vi "SPCSetUpToUserInput.vi"(8 "ErrorIn":errorcluster, 11 "SetUp":string="*SETUP\r\n  SYS_PARA_BEGIN:\r\n  #PR [PR_PDEV,I,2]\r\n  #PR [PR_PPORT,I,2]\r\n  #PR [PR_PWHAT,I,1]\r\n  #PR [PR_PF,B,0]\r\n  #PR [PR_PFNAME,S,C:\\Program Files (x86)\\BH\\SPCM\\IMAGE.PRT]\r\n  #PR [PR_PORIEN,I,1]\r\n  #PR [PR_PEJECT,B,1]\r\n  #PR [PR_PWIDTH,F,100]\r\n  #PR [PR_PHEIGH,F,100]\r\n  #PR [PR_PFULL,B,1]\r\n  #PR [PR_PAUTO,B,1]\r\n  #PR [PR_STP_FN,S,C:\\Users\\frank\\Documents\\BHdata\\SPCM\\STP.CFG]\r\n  #PR [PR_SAVE_T,I,0]\r\n  #PR [PR_SLEEP,I,9]\r\n  #SP [SP_MODE,I,11]\r\n  #SP [SP_CFD_LL,F,-29.411764]\r\n  #SP [SP_CFD_LH,F,5.019608]\r\n  #SP [SP_CFD_ZC,F,-5.2913384]\r\n  #SP [SP_CFD_HF,F,5]\r\n  #SP [SP_SYN_ZC,F,-5.2913384]\r\n  #SP [SP_SYN_FD,I,1]\r\n  #SP [SP_SYN_FQ,F,-50.980392]\r\n  #SP [SP_SYN_HF,F,4]\r\n  #SP [SP_TAC_R,F,5.0033574e-08]\r\n  #SP [SP_TAC_G,I,1]\r\n  #SP [SP_TAC_OF,F,0]\r\n  #SP [SP_TAC_LL,F,0]\r\n  #SP [SP_TAC_LH,F,100]\r\n  #SP [SP_TAC_TC,F,1.2215228e-11]\r\n  #SP [SP_TAC_TD,F,5.0033573e-09]\r\n  #SP [SP_ADC_RE,I,4096]\r\n  #SP [SP_EAL_DE,I,0]\r\n  #SP [SP_NCX,I,1]\r\n  #SP [SP_NCY,I,1]\r\n  #SP [SP_PAGE,I,1]\r\n  #SP [SP_COL_T,F,10]\r\n  #SP [SP_REP_T,F,10]\r\n  #SP [SP_DIS_T,F,1]\r\n  #SP [SP_REPEAT,B,0]\r\n  #SP [SP_STOPT,B,1]\r\n  #SP [SP_OVERFL,C,N]\r\n  #SP [SP_WL_STA,F,500]\r\n  #SP [SP_WL_STO,F,551.09998]\r\n  #SP [SP_WL_STE,F,0.1]\r\n  #SP [SP_EXTST,B,0]\r\n  #SP [SP_STEPS,I,64]\r\n  #SP [SP_OFFSET,F,0]\r\n  #SP [SP_YWIN_N,I,8]\r\n  #SP [SP_XWIN_N,I,8]\r\n  #SP [SP_TWIN_N,I,1]\r\n  #SP [SP_X_EQU,B,1]\r\n  #SP [SP_Y_EQU,B,1]\r\n  #SP [SP_T_EQU,B,1]\r\n  #SP [SP_DITH,I,128]\r\n  #SP [SP_EN_INT,B,0]\r\n  #SP [SP_INCR,I,1]\r\n  #SP [SP_DAES,B,0]\r\n  #SP [SP_SPE_FN,S,c:\\Users\\jannis\\Desktop\\SPC file example\\v1.spc]\r\n  #SP [SP_CYCLES,U,1]\r\n  #SP [SP_DAEC,B,1]\r\n  #SP [SP_MEM_BANK,I,0]\r\n  #SP [SP_DTCOMP,B,0]\r\n  #SP [SP_SCF,I,0]\r\n  #SP [SP_POL_L,I,0]\r\n  #SP [SP_POL_F,I,0]\r\n  #SP [SP_PIX,I,0]\r\n  #SP [SP_LDIV,I,0]\r\n  #SP [SP_ACCUM,B,0]\r\n  #SP [SP_ROUT,B,1792]\r\n  #SP [SP_TAC_EH,F,10]\r\n  #SP [SP_DLIM,I,10240000]\r\n  #SP [SP_PHOT_F,U,473956351]\r\n  #SP [SP_EN_DLIM,B,1]\r\n  #SP [SP_PH_BUF,I,65536]\r\n  #SP [SP_FLB_Y,I,1]\r\n  #SP [SP_FLB_X,I,1]\r\n  #SP [SP_BORD_U,I,1]\r\n  #SP [SP_BORD_L,I,1]\r\n  #SP [SP_POL_P,I,1]\r\n  #SP [SP_PIX_T,F,2.1e-05]\r\n  #SP [SP_PIX_CLK,I,1]\r\n  #SP [SP_TRIGGER,I,16]\r\n  #SP [SP_SCAN_X,I,1]\r\n  #SP [SP_SCAN_Y,I,1]\r\n  #SP [SP_SCAN_RX,I,1]\r\n  #SP [SP_SCAN_RY,I,1]\r\n  #SP [SP_FIF_TYP,I,0]\r\n  #SP [SP_EPX_DIV,I,1]\r\n  #SP [SP_MTCLK,I,0]\r\n  #SP [SP_ADD_SEL,I,0]\r\n  #SP [SP_SXWIN_N,I,1]\r\n  #SP [SP_SYWIN_N,I,1]\r\n  #SP [SP_SX_EQU,B,1]\r\n  #SP [SP_SY_EQU,B,1]\r\n  #SP [SP_ASAVE,I,34]\r\n  #SP [SP_ADC_ZOOM,I,0]\r\n  #SP [SP_FIF_FNO,I,1]\r\n  #SP [SP_FCYCLES,U,1]\r\n  #SP [SP_XY_GAIN,I,1]\r\n  #SP [SP_IMG_X,I,512]\r\n  #SP [SP_IMG_Y,I,512]\r\n  #SP [SP_IMG_RX,I,1]\r\n  #SP [SP_IMG_RY,I,1]\r\n  #SP [SP_MST_CLK,I,0]\r\n  #SP [SP_ADC_DE,I,0]\r\n  #SP [SP_DET_TYP,I,0]\r\n  #SP [SP_X_AXIS,I,0]\r\n  #SP [SP_CH_EN,I,4191231]\r\n  #SP [SP_CH_SL,I,16777215]\r\n  #SP [SP_CH_F1,I,0]\r\n  #SP [SP_CH_F2,I,136314880]\r\n  #DI [DI_SCALE,I,0]\r\n  #DI [DI_MAXCNT,L,2]\r\n  #DI [DI_LBLINE,L,1]\r\n  #DI [DI_BLINE,L,0]\r\n  #DI [DI_GRID,B,1]\r\n  #DI [DI_GCOL_F,I,14737632]\r\n  #DI [DI_GCOL_B,I,16777215]\r\n  #DI [DI_TRACE,I,0]\r\n  #DI [DI_BOD_C,I,32896]\r\n  #DI [DI_2DDIS,I,0]\r\n  #DI [DI_2DTRNO,I,1]\r\n  #DI [DI_3DOFFX,I,3]\r\n  #DI [DI_3DOFFY,I,1]\r\n  #DI [DI_3DINCX,I,0]\r\n  #DI [DI_3DCOL,I,0]\r\n  #DI [DI_3DMODE,I,2]\r\n  #DI [DI_YWIN,I,1]\r\n  #DI [DI_XWIN,I,1]\r\n  #DI [DI_TWIN,I,1]\r\n  #DI [DI_PSTYLE,I,1]\r\n  #DI [DI_PFREQ,I,1]\r\n  #DI [DI_CUR,B,0]\r\n  #DI [DI_RATE,B,1]\r\n  #DI [DI_2DC1,B,1]\r\n  #DI [DI_2DC2,B,1]\r\n  #DI [DI_2DC1C,I,10]\r\n  #DI [DI_2DC2C,I,13]\r\n  #DI [DI_2DC1S,I,0]\r\n  #DI [DI_2DC2S,I,0]\r\n  #DI [DI_3DC1C,I,12]\r\n  #DI [DI_3DC2C,I,14]\r\n  #DI [DI_SIZE,I,0]\r\n  #DI [DI_3DSTYL,I,1]\r\n  #DI [DI_INTCOL,I,1]\r\n  #DI [DI_INTPIX,I,1]\r\n  #DI [DI_COL_NO,I,2]\r\n  #DI [DI_COLMIN,I,0]\r\n  #DI [DI_COLMAX,I,16777215]\r\n  #DI [DI_COL2,I,16711680]\r\n  #DI [DI_COL3,I,255]\r\n  #DI [DI_COL4,I,16776960]\r\n  #DI [DI_COL5,I,65280]\r\n  #DI [DI_HICOL,I,16711680]\r\n  #DI [DI_XREV,B,0]\r\n  #DI [DI_YREV,B,0]\r\n  #DI [DI_DETAIL,B,1]\r\n  #DI [DI_SYWIN,I,1]\r\n  #DI [DI_SXWIN,I,1]\r\n  #DI [DI_ASCALE,I,1]\r\n  SYS_PARA_END:\r\n  TRACE_PARA_BEGIN:\r\n  #TR #0 [1,255,1,1,3,1,1,1]1,1,1]\r\n  #TR #1 [0,16711680,1,1,1,2,1,1]1,1,1]\r\n  #TR #2 [0,65280,1,1,1,3,1,1]1,1,1]\r\n  #TR #3 [0,44,1,1,1,4,1,1]1,1,1]\r\n  #TR #4 [0,16718521,1,1,1,1,1,1]1,1,1]\r\n  #TR #5 [0,16765696,1,1,1,1,1,1]1,1,1]\r\n  #TR #6 [0,22528,1,1,1,1,1,1]1,1,1]\r\n  #TR #7 [0,8684799,1,1,1,1,1,1]1,1,1]\r\n  #TR #8 [0,10374982,1,1,1,1,1,1]1,1,1]\r\n  #TR #9 [0,65473,1,1,1,1,1,1]1,1,1]\r\n  #TR #10 [0,33941,1,1,1,1,1,1]1,1,1]\r\n  #TR #11 [0,123,1,1,1,1,1,1]1,1,1]\r\n  #TR #12 [0,9818959,1,1,1,1,1,1]1,1,1]\r\n  #TR #13 [0,16162524,1,1,1,1,1,1]1,1,1]\r\n  #TR #14 [0,13832959,1,1,1,1,1,1]1,1,1]\r\n  #TR #15 [0,8067690,1,1,1,1,1,1]1,1,1]\r\n  TRACE_PARA_END:\r\n  WIND_PARA_BEGIN:\r\n  #WI #0 *NO *0 [0,0]\r\n  #WI #0 *NO *1 [1,1]\r\n  #WI #0 *NO *2 [2,2]\r\n  #WI #0 *NO *3 [3,3]\r\n  #WI #0 *NO *4 [4,4]\r\n  #WI #0 *NO *5 [5,5]\r\n  #WI #0 *NO *6 [6,6]\r\n  #WI #0 *NO *7 [7,7]\r\n  #WI #1 *NO *0 [0,0]\r\n  #WI #1 *NO *1 [0,0]\r\n  #WI #1 *NO *2 [0,0]\r\n  #WI #1 *NO *3 [0,0]\r\n  #WI #1 *NO *4 [0,0]\r\n  #WI #1 *NO *5 [0,0]\r\n  #WI #1 *NO *6 [0,0]\r\n  #WI #1 *NO *7 [0,0]\r\n  #WI #2 *NO *0 [0,4095]\r\n  #WI #3 *NO *0 [0,0]\r\n  #WI #4 *NO *0 [0,0]\r\n  WIND_PARA_END:\r\n*END") -> (0 "ErrorOut":errorcluster, 1 "adc_resolution_digital":i32, 2 "ADC Resolution Bits":T1=12 items=["-1"=-1, "1"=0, "4"=2, "16"=4, "64"=6, "256"=8, "1024"=10, "4096"=12], 3 "User Input":T2={"tac_range"=50.0, "tac_gain"=3, "tac_offset"=12.0, "tac_limit_high"=96.0, "tac_limit_low"=3.0, "collect_time"=2.0, "sync_threshold"=-71.0, "sync_zc_level"=-5.0, "sync_freq_div"=1, "cfd_limit_low"=-50.0, "cfd_zc_level"=9.8} {"sync_freq_div" items=["1"=1, "2"=2, "4"=4]; "cfd_zc_level" min=-96 max=96 step=0.1 format="%#_3g"; "cfd_limit_low" min=-500 max=0 step=0.1 format="%#_3g"; "sync_zc_level" min=-96 max=96 step=0.1 format="%#_3g"; "sync_threshold" min=-500 max=-20 step=0.1 format="%#_3g"; "tac_limit_low" format="%.3g"; "tac_limit_high" min=0 max=100 step=0.1 format="%.3g"; "collect_time" min=1e-07 max=100000 step=0.001; "tac_offset" min=0 max=100 step=0.1 format="%.4g"; "tac_gain" min=1 max=15 step=1; "tac_range" format="%^#_6g"}, 4 "page":i32, 5 "NoRoutingCh":i32, 6 "dither":i32)   [LabVIEW 2019]
doc: "This VI demonstrates how specific parameters can be entered into an ASCII SetUp-block replacing their default values.\nProvide the Key up to and including the format specifier and trailing comma.\n\ninfo@becker-hickl.com"
uses:
  Examples/Example_Controls/UserInput.ctl
  SPC_Controls/ADCResolution.ctl
panel:
  # "TAC / Time Range"
  # "CFD"
  # "(start)"
  # "SYNC"
  # "(stop)"
  # "range"
  # "gain"
  # "threshold(LL)"
  # "offset"
  # "limit high"
  # "limit low"
  # "zero cross(ZC)"
  # "Collection Time"
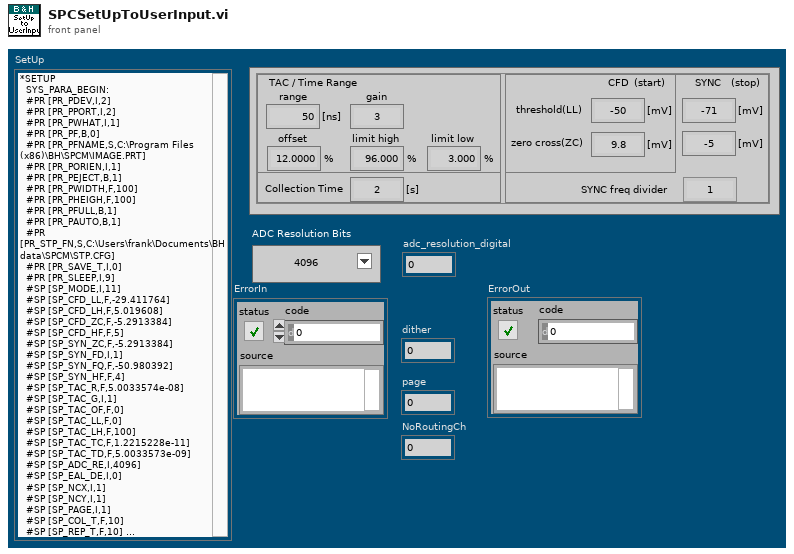
[diagram p1: front panel]
types:
  T1 = typedef "ADCResolution.ctl" = i16
  T2 = typedef "UserInput.ctl" = cluster{"tac_range":sgl, "tac_gain":i16, "tac_offset":sgl, "tac_limit_high":sgl, "tac_limit_low":sgl, "collect_time":sgl, "sync_threshold":sgl, "sync_zc_level":sgl, "sync_freq_div":i16, "cfd_limit_low":sgl, "cfd_zc_level":sgl}
  T3 = cluster{"[0]":dbl, "[1]":dbl, "[2]":dbl, "[3]":dbl, "[4]":dbl, "[5]":dbl, "[6]":dbl, "[7]":dbl, "[8]":dbl, "[9]":dbl, "[10]":dbl}
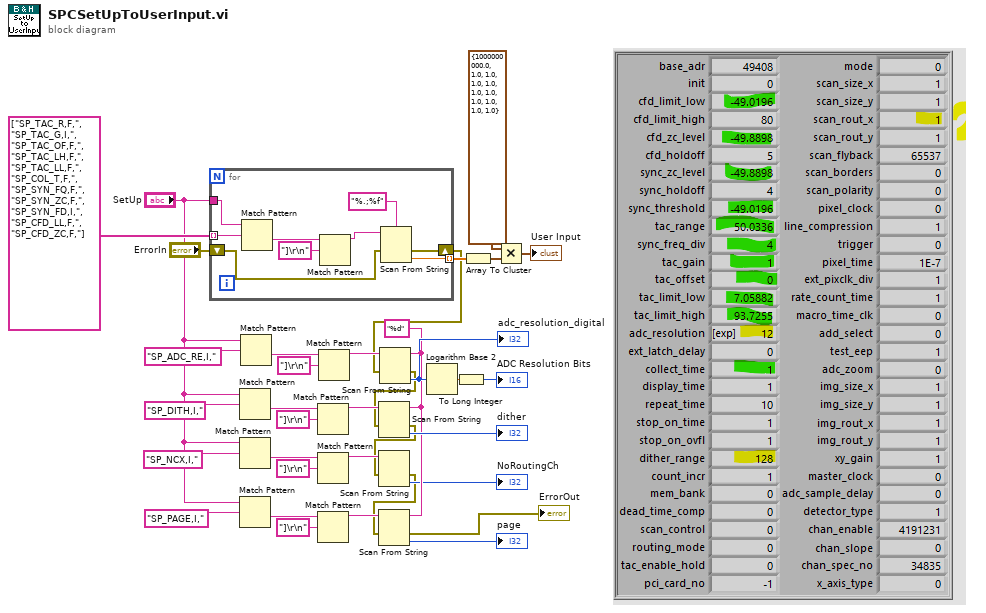
[diagram p0: block diagram]
diagram:
  w13 = "%d" ("format string")
  n1 = for {
    tunnel: string[] ["SP_TAC_R,F,", "SP_TAC_G,I,", "SP_TAC_OF,F,", "SP_TAC_LH,F,", "SP_TAC_LL,F,", "SP_COL_T,F,", "SP_SYN_FQ,F,", "SP_SYN_ZC,F,", "SP_SYN_FD,I,", "SP_CFD_LL,F,", "SP_CFD_ZC,F,"] ("Key") -> [w42] mode=indexing
    tunnel: "SetUp" -> [w41]
    tunnel: [w38] -> w35 mode=indexing
    shift-right: [w37] -> w11
    shift-left: "ErrorIn" -> [w36]
    n2 = Match Pattern(string=w41, regular expression=w42) -> (after substring=w44:string)  [unwired: 1 in, 3 out]
    n3 = Match Pattern(string=w44, regular expression="]\r\n") -> (before substring=w40:string)  [unwired: 1 in, 3 out]
    n4 = Scan From String(format string="%.;%f", input string=w40, error in=w36) -> (error out=w37:errorcluster, output 1=w38:dbl)  [unwired: 2 in, 2 out]
  }
  n5 = Match Pattern(string="SetUp", regular expression="SP_DITH,I," ("Key")) -> (after substring=w22:string)  [unwired: 1 in, 3 out]
  n6 = Match Pattern(string="SetUp", regular expression="SP_NCX,I," ("Key")) -> (after substring=w5:string)  [unwired: 1 in, 3 out]
  n7 = Match Pattern(string="SetUp", regular expression="SP_PAGE,I," ("Key")) -> (after substring=w15:string)  [unwired: 1 in, 3 out]
  n8 = Match Pattern(string="SetUp", regular expression="SP_ADC_RE,I," ("Key")) -> (after substring=w28:string)  [unwired: 1 in, 3 out]
  n9 = Match Pattern(string=w22, regular expression="]\r\n") -> (before substring=w20:string)  [unwired: 1 in, 3 out]
  n10 = Match Pattern(string=w5, regular expression="]\r\n") -> (before substring=w7:string)  [unwired: 1 in, 3 out]
  n11 = Match Pattern(string=w15, regular expression="]\r\n") -> (before substring=w17:string)  [unwired: 1 in, 3 out]
  n12 = Match Pattern(string=w28, regular expression="]\r\n") -> (before substring=w30:string)  [unwired: 1 in, 3 out]
  n13 = Scan From String(format string=w13, input string=w30, error in=w11) -> (error out=w10:errorcluster, output 1=w25:i32)  [unwired: 2 in, 2 out]
  "adc_resolution_digital" <- w25
  n14 = Scan From String(format string=w13, input string=w20, error in=w10) -> (error out=w3:errorcluster, output 1=→"dither":i32)  [unwired: 2 in, 2 out]
  n15 = Scan From String(input string=w7, error in=w3) -> (error out=w2:errorcluster, output 1=→"NoRoutingCh":i32)  [unwired: 3 in, 2 out]
  n16 = Scan From String(format string=w13, input string=w17, error in=w2) -> (error out=→"ErrorOut":errorcluster, output 1=→"page":i32)  [unwired: 2 in, 2 out]
  n17 = Logarithm Base 2(1:w25) -> (0:w26:dbl)
  n18 = To Long Integer(number=w26) -> (32bit integer=→"ADC Resolution Bits":i32)
  n19 = Array To Cluster(array=w35) -> (cluster=w34:T3)
  n20 = Multiply(x=T3 {"[0]"=1000000000.0, "[1]"=1.0, "[2]"=1.0, "[3]"=1.0, "[4]"=1.0, "[5]"=1.0, "[6]"=1.0, "[7]"=1.0, "[8]"=1.0, "[9]"=1.0, "[10]"=1.0}, y=w34) -> (x*y=→"User Input":T3)
